vi "Temperature Limit.vi"() -> ()   [LabVIEW 2015]
doc: "This VI simulates the acquisition of temperature, graphs the temperature, and notifies the user if the temperature is over the limit."
panel:
  in  "Start":bool
  in  "Delta t (ms)":i32(slide)=400 scale=50.0..500.0
  in  "Stop":bool
  in  "High Limit":dbl=28.0 format="%.2f"
  out "Temperature":cluster{"Temperature":dbl, "High Limit":dbl}(graph)={"Temperature"=85.88749999999999, "High Limit"=80.0}
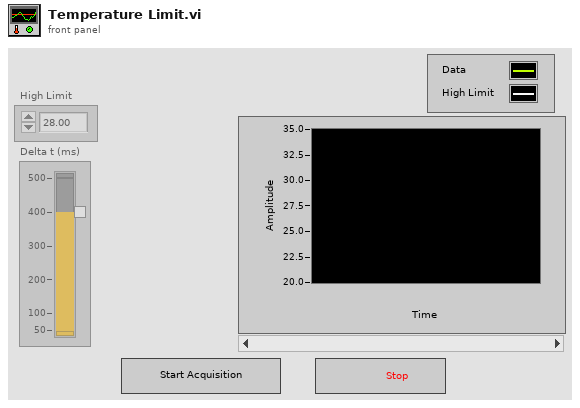
[diagram p1: front panel]
types:
  T1 = enum8{"Enabled", "Disabled", "Disabled and Grayed Out"}
  T2 = cluster{"Temperature Value":dbl, "High Limit":dbl}
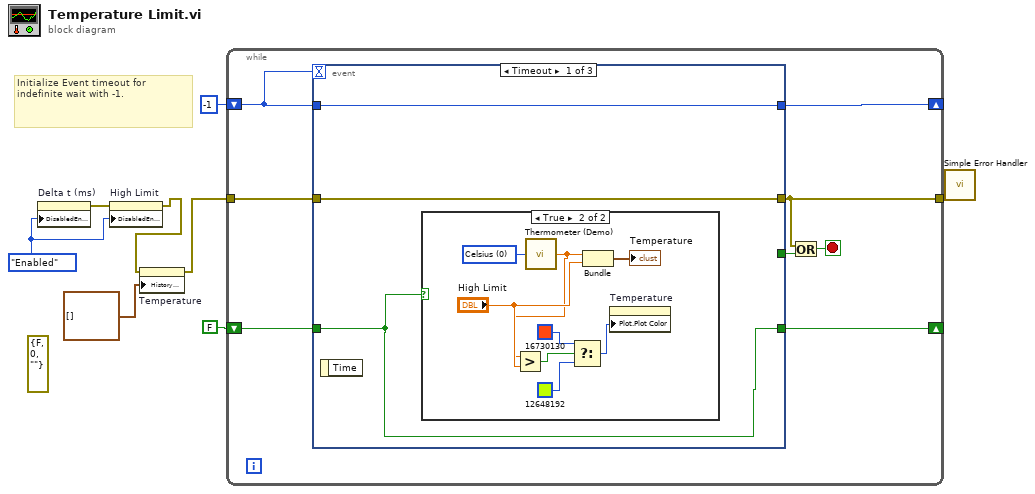
[diagram p0: block diagram]
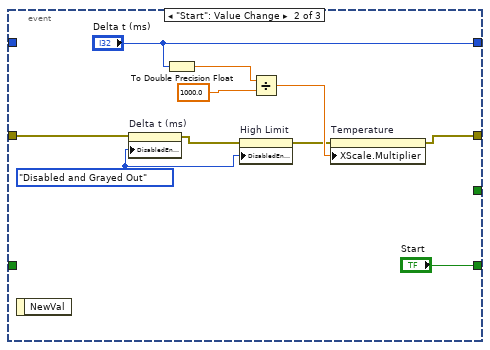
[diagram p3: hidden frame]
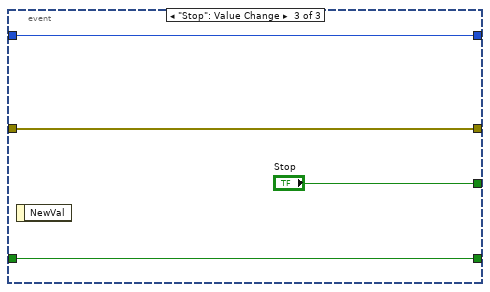
[diagram p4: hidden frame]
diagram:
  w4 = T1."Enabled" ("Disabled")
  (unwired) errorcluster {"status"=FALSE, "code"=0, "source"=""} ("error out")
  # "Initialize Event timeout for indefinite wait with -1."
  n1 = property on="Delta t (ms)" class="Slide (strict)"("DisabledEnum"=w4) -> (error out=w5:errorcluster)  [unwired: 2 in, 1 out]
  n2 = property on="High Limit" class="DigNum (strict)"(error in=w5, "DisabledEnum"=w4) -> (error out=w2:errorcluster)  [unwired: 1 in, 1 out]
  n3 = property on="Temperature" class="WFChart (strict)"(error in=w2, "History Data"=cluster{"Temperature":dbl, "High Limit":dbl}[] []) -> (error out=w1:errorcluster)  [unwired: 1 in, 1 out]
  n4 = while {
    tunnel: w1 -> [w16]
    tunnel: [w14] -> w7
    shift-right: [w12] -> _
    shift-left: FALSE ("Start") -> [w11]
    shift-right: [w10] -> _
    shift-left: -1 ("Delta t (ms)") -> [w9]
    stop <- w15 stop-if-true
    n5 = event shown="[0] Timeout" {
      selector: _ -> [_ _ _]
      dyn-events: _ -> [_ _ _]
      timeout: w9 -> [_ _ _]
      tunnel: [_ _ "Stop"] -> w13
      tunnel: w16 -> [w18 w36 w38]
      tunnel: [w18 w34 w38] -> w14
      tunnel: [w17 "Start" w40] -> w12
      tunnel: w11 -> [w17 _ w40]
      tunnel: [w19 "Delta t (ms)" w39] -> w10
      tunnel: w9 -> [w19 _ w39]
      event Timeout {
        n6 = event-data() -> ()  [unwired: 1 in, 1 out]
        n7 = case shown="True" w17 {
          frame False {
          }
          frame True {
            w26 = u16 0 items=["Celsius", "Fahrenheit"] ("Units (0: Celsius)")
            n8 = call "Thermometer (Demo).vi"("Units (0: Celsius)"=w26) -> ("Temperature Value"=w20:dbl)
            n9 = Greater?(x=w20, y="High Limit") -> (0:w22:bool)
            n10 = Select(t=u32 16730130, s=w22, f=u32 12648192) -> (s? t:f=w23:u32)
            n11 = Bundle("Temperature Value"=w20, "High Limit"="High Limit") -> (→"Temperature":T2)  [unwired: 1 in]
            n12 = property on="Temperature" class="WFChart (strict)"("Plot.Plot Color"=w23) -> ()  [unwired: 2 in, 2 out]
          }
        }
      }
      event "Start": Value Change {
        w29 = T1."Disabled and Grayed Out" ("Disabled")
        n13 = event-data() -> ()  [unwired: 1 in, 1 out]
        n14 = property on="Delta t (ms)" class="Slide (strict)"(error in=w36, "DisabledEnum"=w29) -> (error out=w35:errorcluster)  [unwired: 1 in, 1 out]
        n15 = To Double Precision Float(number="Delta t (ms)") -> (double precision float=w32:dbl)
        n16 = property on="High Limit" class="DigNum (strict)"(error in=w35, "DisabledEnum"=w29) -> (error out=w28:errorcluster)  [unwired: 1 in, 1 out]
        n17 = Divide(x=w32, y=1000.0) -> (x/y=w30:dbl)
        n18 = property on="Temperature" class="WFChart (strict)"(error in=w28, "XScale.Multiplier"=w30) -> (error out=w34:errorcluster)  [unwired: 1 in, 1 out]
      }
      event "Stop": Value Change {
        n19 = event-data() -> ()  [unwired: 1 in, 1 out]
      }
    }
    n20 = Or(x=w14, y=w13) -> (x .or. y?=w15:bool)
  }
  n21 = call <vilib>:"Simple Error Handler.vi"("error in (no error)"=w7) -> ()  [unwired: 4 in, 5 out]
